vi "Configure Trigger (CAN - Identifier Or Data).vi"(0 "VISA resource name":refnum<visa-resource-name>, 1 "Data Threshold (0.0V)":dbl, 2 "Nominal Bit Rate(1MB)":dbl=1000000.0, 3 "CAN Format (0:Standard)":u16(ring) items=["Standard", "Extended"], 5 "Source (0:Channel1)":u16(ring) items=["Channel1", "Channel2", "Channel3", "Channel4"], 7 "Signal Type (0:Differential)":u16(ring) items=["Differential", "CAN + H", "CAN - L", "TX", "RX"], 9 "Trigger Condition (2:Identifier)":u16(ring)=2 items=["Identifier"=2, "Data"=3, "Identifier And Data"=4], 11 "error in (no error)":errorcluster, 12 "Data Direction(0:Either)":u16(ring) items=["Either", "Read", "Write"], 13 "Data Value":string, 14 "Identifier Vale":string caption="Identifier Value") -> (4 "VISA resource name out":refnum<visa-resource-name>, 15 "error out":errorcluster)   [LabVIEW 2011, in "Tektronix 7000 Series.lvlib"]
doc: "Configures CAN trigger settings(Identifier, Data , Identifier and Data) for an oscilloscope.A trigger occurs when a Controller Area Network frame signal is found.\n\nOnly DPO7000 series oscilloscopes Support CAN Trigger."
uses:
  Tektronix 7000 Series.lvlib
panel:
  # "msb"
  # "lsb"
  # "lsb"
  # "msb"
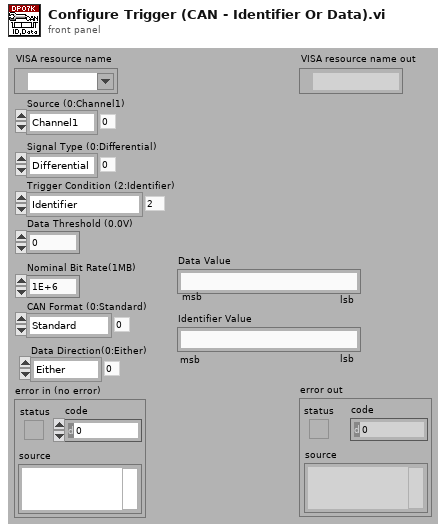
[diagram p1: front panel]
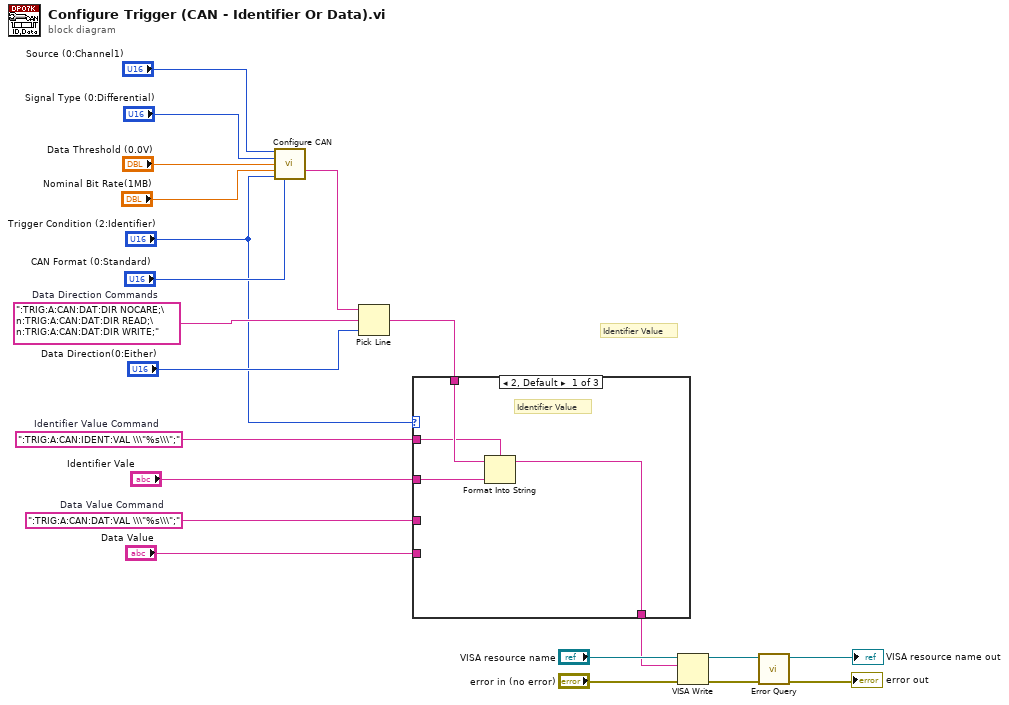
[diagram p0: block diagram]
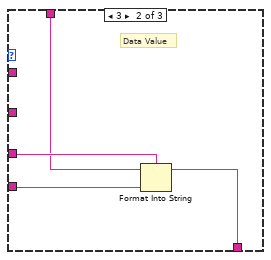
[diagram p2: hidden frame]
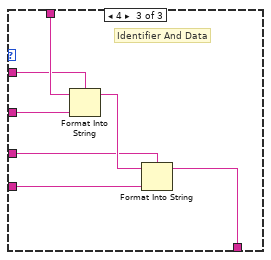
[diagram p3: hidden frame]
diagram:
  w9 = ":TRIG:A:CAN:DAT:VAL \\\"%s\\\";"  # Data Value Command
  w11 = ":TRIG:A:CAN:IDENT:VAL \\\"%s\\\";"  # Identifier Value Command
  w15 = ":TRIG:A:CAN:DAT:DIR NOCARE;\n:TRIG:A:CAN:DAT:DIR READ;\n:TRIG:A:CAN:DAT:DIR WRITE;"  # Data Direction Commands
  # "Identifier Value"
  n1 = call "Configure CAN.vi"("Source (0:Channel1)"="Source (0:Channel1)", "Signal Type (0:Differential)"="Signal Type (0:Differential)", "Data Threshold (0.0V)"="Data Threshold (0.0V)", "Nominal Bit Rate (1MB)"="Nominal Bit Rate(1MB)", "Trigger Condition (0:Start)"="Trigger Condition (2:Identifier)", "CAN Format (0:Standard)"="CAN Format (0:Standard)") -> ("Output String"=w16:string)  [unwired: 9 in]
  n2 = Pick Line(string ("")=w16, multi-line string=w15, line index="Data Direction(0:Either)") -> (output string=w12:string)
  n3 = case shown="2, Default" "Trigger Condition (2:Identifier)" {
    tunnel: w12 -> [w25 w27 w35]
    tunnel: w11 -> [w24 _ w34]
    tunnel: "Identifier Vale" -> [w23 _ w36]
    tunnel: w9 -> [_ w28 w32]
    tunnel: "Data Value" -> [_ w29 w31]
    tunnel: [w22 w26 w30] -> w1
    frame 2, Default {
      # "Identifier Value"
      n4 = Format Into String(format string=w24, initial string=w25, w23) -> (resulting string=w22:string)  [unwired: 1 in, 1 out]
    }
    frame 3 {
      # "Data Value"
      n5 = Format Into String(format string=w28, initial string=w27, w29) -> (resulting string=w26:string)  [unwired: 1 in, 1 out]
    }
    frame 4 {
      # "Identifier And Data"
      n6 = Format Into String(format string=w34, initial string=w35, w36) -> (resulting string=w33:string)  [unwired: 1 in, 1 out]
      n7 = Format Into String(format string=w32, initial string=w33, w31) -> (resulting string=w30:string)  [unwired: 1 in, 1 out]
    }
  }
  n8 = VISA Write(VISA resource name="VISA resource name", write buffer=w1, error in (no error)="error in (no error)") -> (VISA resource name out=w7:refnum<visa-resource-name>, error out=w6:errorcluster)  [unwired: 1 out]
  n9 = call "Error Query.vi"("error in (no error)"=w6, "VISA resource name"=w7) -> ("error out"=→"error out":errorcluster, "VISA resource name out"=→"VISA resource name out":refnum<visa-resource-name>)  [unwired: 6 in, 2 out]
